vi "Init.vi"(8 "error in (no error)":errorcluster, 10 "Address":string, 11 "HRS_Spectrometer in":refnum<class "HRS_Spectrometer.lvclass">) -> (0 "error out":errorcluster, 3 "HRS_Spectrometer out":refnum<class "HRS_Spectrometer.lvclass">)   [LabVIEW 2023, in "HRS_Spectrometer.lvlib" / "HRS_Spectrometer.lvclass"]
uses:
  HRS_Spectrometer.lvclass
  HRS_Spectrometer.lvclass/HRS_Spectrometer.ctl
  Cameras_LV/InitDeinitComm Messages/InitDone Msg/InitDone Msg.lvclass
  <vilib>/ActorFramework/Actor/Actor.lvclass
  <vilib>/Instr/_visa.llb/Select Event Type.ctl
  Applications/National Instruments/LabVIEW 2023 64-bit/vi.lib/ActorFramework/Actor/Actor.lvclass
  Users/alexandrosspiliotis/Documents/LV_DAQ_Project/Spectrometer_HRS_LV/HRS_Spectrometer/HRS_Spectrometer/HRS_Spectrometer.lvclass
  Users/alexandrosspiliotis/Documents/LV_DAQ_Project/Spectrometer_HRS_LV/Spectrometer.lvclass
  Users/alexandrosspiliotis/Documents/LV_DAQ_Project/Cameras_LV/InitDeinit/InitDeinit.lvclass
panel:
  in  "Address cluster":T1
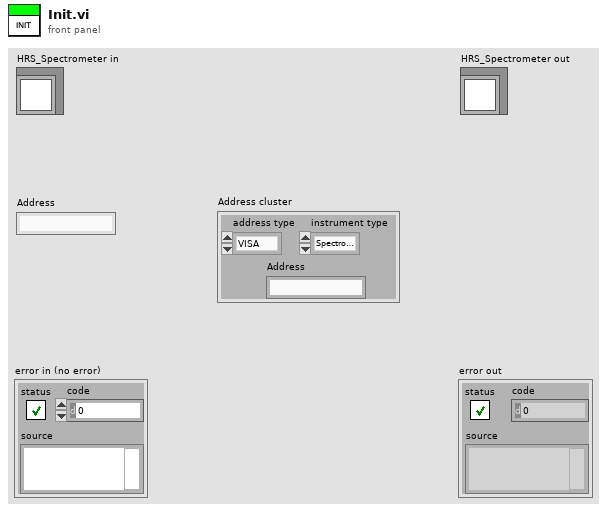
[diagram p1: front panel]
types:
  T1 = cluster{"address type":enum16{"VISA", "Index"}, "Address":string, "instrument type":enum16{"Spectrometer", "Camera", "Stepper"}}
  T2 = typedef "Select Event Type.ctl" = u32
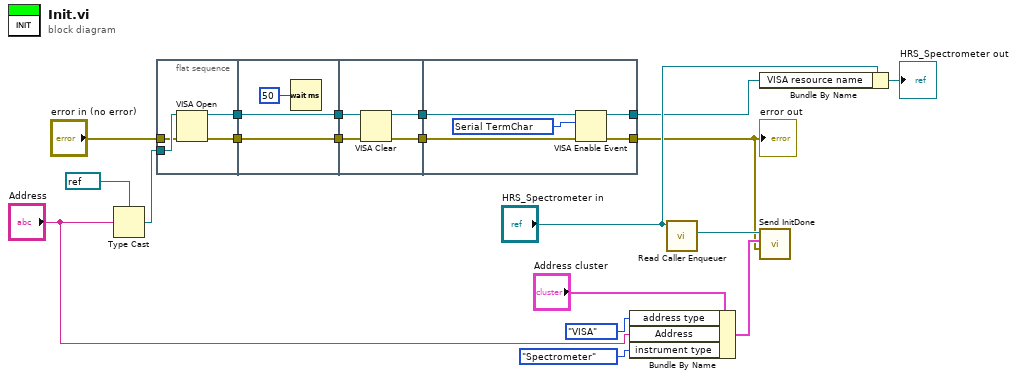
[diagram p0: block diagram]
diagram:
  n1 = Type Cast(type=refnum<visa-resource-name> refnum ("VISA resource name"), x="Address") -> (*(type *) &x=w18:refnum<visa-resource-name>)
  n2 = flat-sequence {
    tunnel: w18 -> [w23]
    tunnel: "error in (no error)" -> [w22]
    tunnel: [w21] -> w16
    tunnel: [w20] -> w14
    tunnel: w16 -> [w25]
    tunnel: [w25] -> w15
    tunnel: w14 -> [w24]
    tunnel: [w24] -> w13
    tunnel: w15 -> [w30]
    tunnel: w13 -> [w29]
    tunnel: [w28] -> w2
    tunnel: [w27] -> w1
    tunnel: [w33] -> w5
    tunnel: [w31] -> w7
    tunnel: w2 -> [w32]
    tunnel: w1 -> [w34]
    frame #0 {
      n3 = VISA Open(error in (no error)=w22, VISA resource name=w23) -> (VISA resource name=w21:refnum<visa-resource-name>, error out=w20:errorcluster)  [unwired: 3 in]
    }
    frame #1 {
      n4 = Wait (ms)(milliseconds to wait=u32 50) -> ()  [unwired: 1 out]
    }
    frame #2 {
      n5 = VISA Clear(VISA resource name=w30, error in (no error)=w29) -> (VISA resource name out=w27:refnum<visa-resource-name>, error out=w28:errorcluster)
    }
    frame #3 {
      w35 = T2 1073684516 items=["Service Request"=1073684491, "Trigger"=3221168138, "Clear"=1073684493, "VXI Signal"=1073684512, "VXI/VME Interrupt"=3221168161, "VXI/VME Sysfail"=1073684509, "VXI/VME Sysreset"=1073684510, "GPIB CIC"=1073684498, "GPIB Talk"=1073684499, "GPIB Listen"=1073684500, "PXI Interrupt"=1073684514, "Serial Break"=1073684515, "Serial TermChar"=1073684516, "Serial CTS"=1073684521, "Serial DSR"=1073684522, "Serial DCD"=1073684524, "Serial RI"=1073684526, "Serial Character"=1073684533, "USB Interrupt"=1073684535, "All Enabled"=1073709055] ("Event Type")
      n6 = VISA Enable Event(8:w32, 10:w35, 11:w34) -> (0:w31:errorcluster, 3:w33:refnum<visa-resource-name>)  [unwired: 1 in]
    }
  }
  n7 = Bundle By Name(cluster="Address cluster", "address type"=enum16{"VISA", "Index"}."VISA", "Address"="Address", "instrument type"=enum16{"Spectrometer", "Camera", "Stepper"}."Spectrometer") -> (w10:T1)
  n8 = call <vilib>:"Read Caller Enqueuer.vi"("Actor"="HRS_Spectrometer in") -> ("Caller Enqueuer"=w12:refnum<class "Message Enqueuer.lvclass">)  [unwired: 10 in]
  n9 = Bundle By Name(cluster="HRS_Spectrometer in", "VISA resource name"=w5) -> (→"HRS_Spectrometer out":refnum<class "HRS_Spectrometer.lvclass">)
  n10 = call "Send InitDone.vi"("instr error"=w7, "Address"=w10, "Message Enqueuer"=w12) -> ()  [unwired: 7 in, 2 out]
  "error out" <- w7
